vi "onHttpPatch (Buffer).vi"(8 "error in":errorcluster, 10 "httpRequest":refnum<class "httpRequest.lvclass">, 11 "advanced-http-client in":refnum<class "advanced-http-client.lvclass">) -> (0 "error out":errorcluster, 2 "httpResponse":refnum<class "httpResponse.lvclass">, 3 "advanced-http-client out":refnum<class "advanced-http-client.lvclass">)   [LabVIEW 2020, in "HttpClient.NiAdvanced.lvlib" / "advanced-http-client.lvclass"]
uses:
  advanced-http-client.lvclass
  advanced-http-client.lvclass/advanced-http-client.ctl
  <vilib>/NI/Advanced HTTP Client/Session.lvclass
  <vilib>/NI/Advanced HTTP Client/PATCH (Buffer).vi
  http-client-pkg/httpRequest/httpRequest.lvclass
  http-client-pkg/httpResponse/httpResponse.lvclass
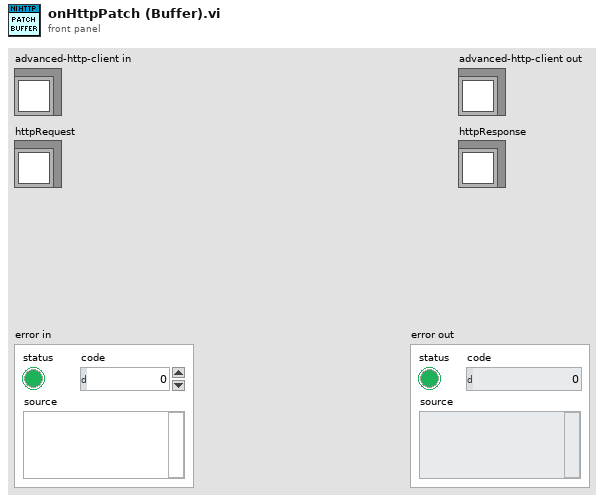
[diagram p1: front panel]
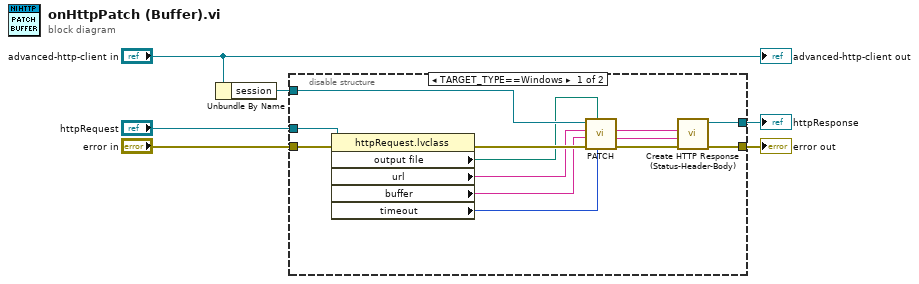
[diagram p0: block diagram]
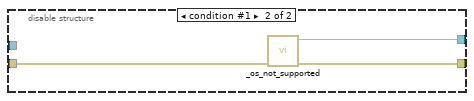
[diagram p2: hidden frame]
diagram:
  n1 = Unbundle By Name("advanced-http-client in") -> ("session"=w5:refnum<class "Session.lvclass">)
  n2 = disable-structure shown="TARGET_TYPE==Windows" {
    disable-tunnel: w5 -> [w19 _]
    disable-tunnel: "error in" -> [w16 w22]
    disable-tunnel: [w9 w21] -> w3
    disable-tunnel: "httpRequest" -> [w18 _]
    disable-tunnel: [w7 w20] -> w1
    frame condition #0 (active) {
      n3 = property class="httpRequest.lvclass"(reference=w18, error in=w16) -> (error out=w17:errorcluster, "output file"=w15:path, "url"=w14:string, "buffer"=w13:string, "timeout"=w12:i32)  [unwired: 1 out]
      n4 = call-poly <vilib>:"PATCH.vi"("timeout"=w12, "output file"=w15, "error in"=w17, "buffer"=w13, "url"=w14, "session in"=w19) -> ("error out"=w10:errorcluster, "body"=w11:string, "headers"=w8:string)  [unwired: 1 in, 2 out]
      n5 = call "Create HTTP Response (Status-Header-Body).vi"("error in"=w10, "body"=w11, "Headers w/ status line(s)"=w8) -> ("error out"=w9:errorcluster, "httpResponse out"=w7:refnum<class "httpResponse.lvclass">)  [unwired: 7 in]
    }
    frame condition #1 {
      n6 = call "_os_not_supported.vi"("error in (no error)"=w22) -> ("error out"=w21:errorcluster, "httpResponse"=w20:refnum<class "httpResponse.lvclass">)  [unwired: 9 in]
    }
  }
  "error out" <- w3
  "httpResponse" <- w1
  "advanced-http-client out" <- "advanced-http-client in"
